vi "Read HIJ Vision Camera App.vi"(8 "error in (no error)":errorcluster, 11 "HIJ Vision Launcher in":refnum<class "HIJ Vision Launcher.lvclass">) -> (0 "error out":errorcluster, 2 "ViewableActor.lvlib:ViewableActor.lvclass":refnum<class "ViewableActor.lvclass">, 3 "HIJ Vision Launcher out":refnum<class "HIJ Vision Launcher.lvclass">)   [LabVIEW 2014, in "HIJ Vision Launcher.lvlib" / "HIJ Vision Launcher.lvclass"]
uses:
  HIJ Vision Launcher.lvclass
  Shared Code/Viewable Actor/ViewableActor/ViewableActor.lvclass
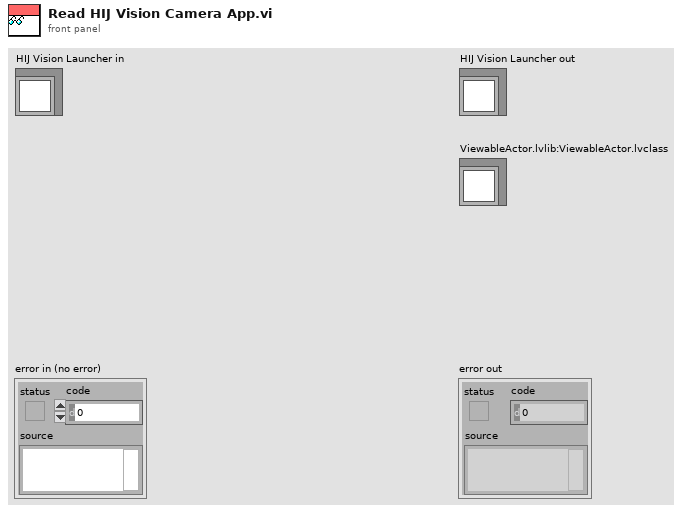
[diagram p1: front panel]
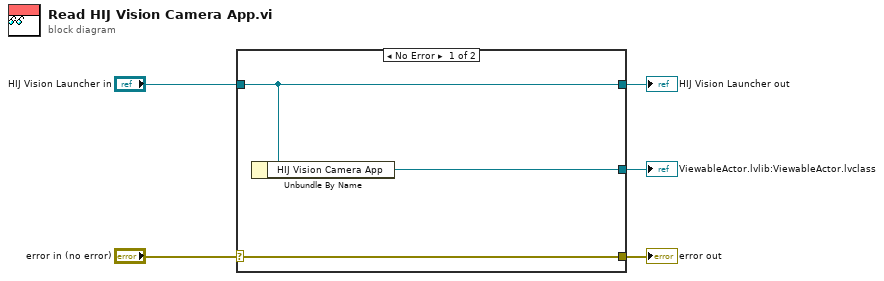
[diagram p0: block diagram]
diagram:
  n1 = case shown="No Error" "error in (no error)" {
    selector: "error in (no error)" -> [w8 w9]
    tunnel: [w8 w9] -> w4
    tunnel: [w7 w10] -> w2
    tunnel: "HIJ Vision Launcher in" -> [w7 w10]
    tunnel: [w6 _] -> w1
    frame No Error {
      n2 = Unbundle By Name(w7) -> ("HIJ Vision Camera App"=w6:refnum<class "ViewableActor.lvclass">)
    }
    frame Error {
    }
  }
  "error out" <- w4
  "HIJ Vision Launcher out" <- w2
  "ViewableActor.lvlib:ViewableActor.lvclass" <- w1
